vi "Check Arduino Port_MI.vi"(8 "error in (no error)":errorcluster) -> (0 "error out":errorcluster, 1 "Instrument Name Array":string[](array[string]), 2 "Visa Instrument list":string[](array[string]), 3 "VISA Refnum out":refnum<visa-resource-name>)   [LabVIEW 2019, in "Machine Interface.lvclass"]
uses:
  Machine Interface.lvclass
  <vilib>/Instr/_visa.llb/VISA Find Search Mode.ctl
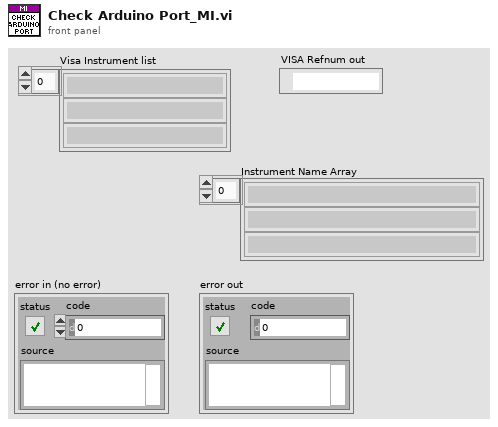
[diagram p1: front panel]
types:
  T1 = typedef "VISA Find Search Mode.ctl" = u32
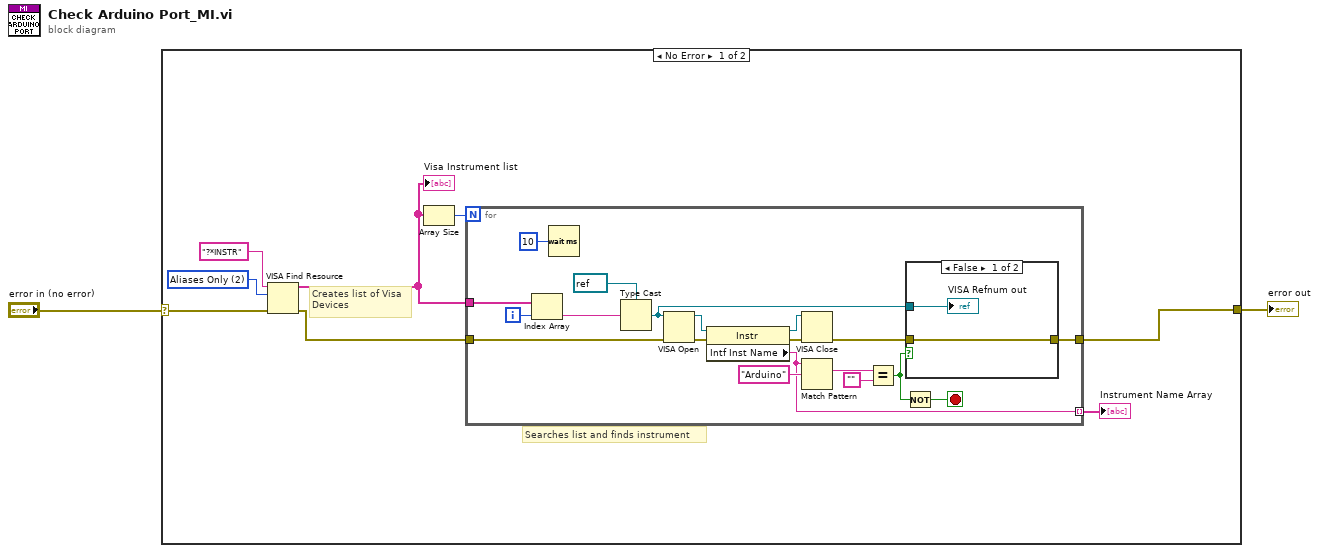
[diagram p0: block diagram]
diagram:
  n1 = case shown="No Error" "error in (no error)" {
    selector: "error in (no error)" -> [w4 w33]
    tunnel: [w10 w33] -> w2
    frame No Error {
      w8 = T1 2 items=["Canonical Names Only"=0, "Aliases Only"=2, "Include Matching Aliases"=3, "Include All Aliases"=4] ("Search Mode")
      # "Searches list and finds instrument"
      # "Creates list of Visa \nDevices"
      n2 = VISA Find Resource(8:w4, 10:w8, 11:"?*INSTR" ("expression (\"?*\")")) -> (0:w3:errorcluster, 3:w7:string[])  [unwired: 1 out]
      "Visa Instrument list" <- w7
      n3 = Array Size(array=w7) -> (size(s)=w5:i32)
      n4 = for {
        N: w5 -> [_]
        tunnel: w7 -> [w29]
        tunnel: [w25] -> w6 mode=indexing
        tunnel: [w12] -> w10
        tunnel: w3 -> [w11]
        i -> [w27]
        stop <- w16 stop-if-true
        n5 = Index Array(array=w29, index=w27) -> (element=w21:string)
        n6 = Wait (ms)(milliseconds to wait=u32 10) -> ()  [unwired: 1 out]
        n7 = Type Cast(type=refnum<visa-resource-name> refnum ("VISA resource name"), x=w21) -> (*(type *) &x=w17:refnum<visa-resource-name>)
        n8 = VISA Open(error in (no error)=w11, VISA resource name=w17) -> (VISA resource name=w28:refnum<visa-resource-name>, error out=w23:errorcluster)  [unwired: 3 out]
        n9 = property class="Instr"(reference=w28, error in=w23) -> (reference out=w18:refnum<visa-resource-name>, error out=w14:errorcluster, "Intf Inst Name"=w25:string)
        n10 = VISA Close(VISA resource name=w18, error in (no error)=w14) -> (error out=w13:errorcluster)
        n11 = Match Pattern(string=w25, regular expression="Arduino" ("Unique Identifier")) -> (match substring=w20:string)  [unwired: 4 out]
        n12 = Equal?(x=w20, y="") -> (x = y?=w15:bool)
        n13 = Not(x=w15) -> (.not. x?=w16:bool)
        n14 = case shown="False" w15 {
          tunnel: w17 -> [w31 _]
          tunnel: w13 -> [w30 w32]
          tunnel: [w30 w32] -> w12
          frame False {
            "VISA Refnum out" <- w31
          }
          frame True {
          }
        }
      }
      "Instrument Name Array" <- w6
    }
    frame Error {
    }
  }
  "error out" <- w2
